vi "PDU Init.vi"(8 "error in (no error)":errorcluster, 10 "Name":string, 11 "Power Distribution in":refnum<class "Power Distribution.lvclass">) -> (0 "error out":errorcluster, 3 "Power Distribution out":refnum<class "Power Distribution.lvclass">)   [LabVIEW 2022 SP3, in "Power Distribution.lvclass"]
uses:
  Power Distribution.lvclass
  Power Distribution.lvclass/Power Distribution.ctl
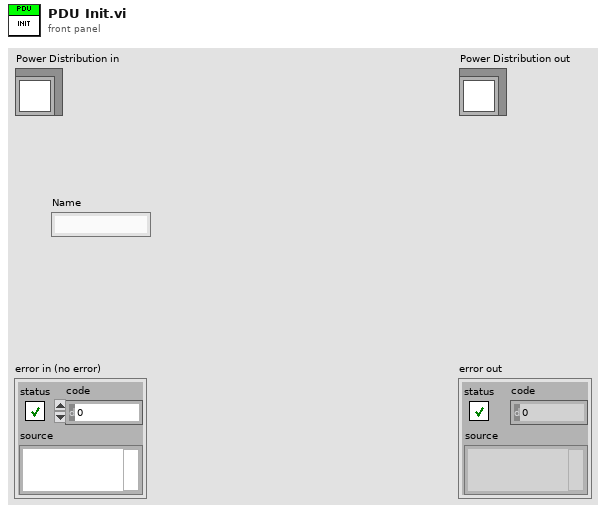
[diagram p1: front panel]
types:
  T1 = typedef "Power Distribution.lvclass/PDU typedef Settings.ctl" = cluster{"Names":string[]}
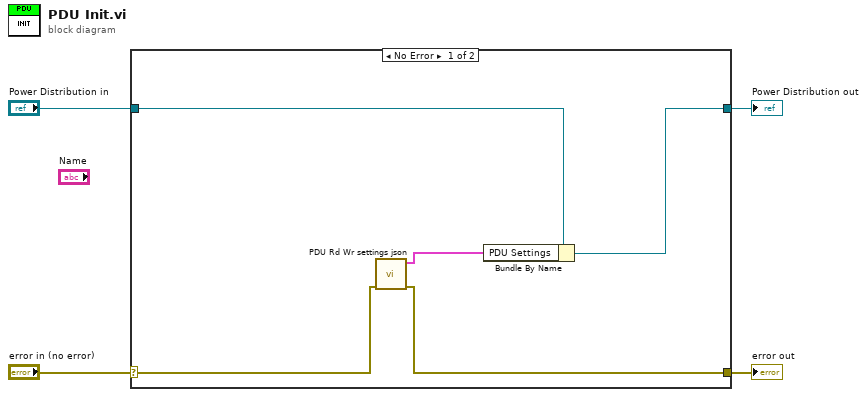
[diagram p0: block diagram]
diagram:
  n1 = case shown="No Error" "error in (no error)" {
    selector: "error in (no error)" -> [w9 w11]
    tunnel: [w8 w11] -> w3
    tunnel: [w6 w10] -> w1
    tunnel: "Power Distribution in" -> [w5 w10]
    frame No Error {
      n2 = call "PDU Rd Wr settings json.vi"("error in (no error)"=w9) -> ("error out"=w8:errorcluster, "PDU Settings"=w7:T1)  [unwired: 9 in]
      n3 = Bundle By Name(cluster=w5, "PDU Settings"=w7) -> (w6:refnum<class "Power Distribution.lvclass">)
    }
    frame Error {
    }
  }
  "error out" <- w3
  "Power Distribution out" <- w1
